vi "Func-엑셀 데이터를 그래프로 출력.vi"() -> ()   [LabVIEW 2015] (continued)
\t33.031\n30.25\t29.31\t33.06\n30.333\t29.34\t33.08\n30.417\t29.38\t33.1\n30.5\t29.41\t33.128\n30.583\t29.44\t33.149\n30.667\t29.49\t33.181\n30.75\t29.52\t33.201\n30.833\t29.58\t33.234\n30.917\t29.64\t33.257\n31\t29.69\t33.277\n31.083\t29.76\t33.311\n31.167\t29.83\t33.344\n31.25\t29.9\t33.378\n31.333\t29.99\t33.4\n31.417\t30.07\t33.435\n31.5\t30.16\t33.464\n31.583\t30.25\t33.499\n31.667\t30.34\t33.531\n31.75\t30.43\t33.566\n31.833\t30.52\t33.598\n31.917\t30.61\t33.637\n32\t30.7\t33.664\n32.083\t30.78\t33.702\n32.167\t30.87\t33.738\n32.25\t30.96\t33.777\n32.333\t31.05\t33.805\n32.417\t31.14\t33.841\n32.5\t31.22\t33.877\n32.583\t31.31\t33.921\n32.667\t31.39\t33.946\n32.75\t31.48\t33.992\n32.833\t31.56\t34.028\n32.917\t31.64\t34.072\n33\t31.72\t34.12\n33.083\t31.8\t34.156\n33.167\t31.89\t34.186\n33.25\t31.96\t34.234\n33.333\t32.04\t34.273\n33.417\t32.13\t34.311\n33.5\t32.21\t34.349\n33.583\t32.29\t34.399\n33.667\t32.38\t34.444\n33.75\t32.46\t34.48\n33.833\t32.54\t34.524\n33.917\t32.62\t34.567\n34\t32.7\t34.611\n34.083\t32.78\t34.659\n34.167\t32.86\t34.71\n34.25\t32.95\t34.745\n34.333\t33.03\t34.793\n34.417\t33.1\t34.843\n34.5\t33.19\t34.884\n34.583\t33.27\t34.936\n34.667\t33.34\t34.972\n34.75\t33.43\t35.024\n34.833\t33.51\t35.072\n34.917\t33.6\t35.12\n35\t33.68\t35.169\n35.083\t33.76\t35.219\n35.167\t33.84\t35.261\n35.25\t33.91\t35.317\n35.333\t34\t35.361\n35.417\t34.08\t35.414\n35.5\t34.16\t35.466\n35.583\t34.24\t35.516\n35.667\t34.32\t35.568\n35.75\t34.4\t35.617\n35.833\t34.48\t35.672\n35.917\t34.56\t35.721\n36\t34.64\t35.772\n36.083\t34.72\t35.825\n36.167\t34.81\t35.89\n36.25\t34.91\t35.929\n36.333\t34.98\t35.979\n36.417\t35.06\t36.035\n36.5\t35.15\t36.089\n36.583\t35.23\t36.138\n36.667\t35.31\t36.195\n36.75\t35.4\t36.259\n36.833\t35.47\t36.321\n36.917\t35.56\t36.369\n37\t35.64\t36.425\n37.083\t35.72\t36.47\n37.167\t35.81\t36.541\n37.25\t35.89\t36.585\n37.333\t35.96\t36.646\n37.417\t36.05\t36.697\n37.5\t36.13\t36.768\n37.583\t36.21\t36.809\n37.667\t36.3\t36.873\n37.75\t36.37\t36.934\n37.833\t36.46\t36.986\n37.917\t36.54\t37.046\n38\t36.62\t37.108\n38.083\t36.71\t37.157\n38.167\t36.79\t37.223\n38.25\t36.87\t37.283\n38.333\t36.96\t37.336\n38.417\t37.05\t37.39\n38.5\t37.13\t37.46\n38.583\t37.21\t37.511\n38.667\t37.3\t37.579\n38.75\t37.38\t37.633\n38.833\t37.47\t37.689\n38.917\t37.53\t37.751\n39\t37.62\t37.814\n39.083\t37.7\t37.879\n39.167\t37.78\t37.939\n39.25\t37.86\t37.999\n39.333\t37.95\t38.054\n39.417\t38.04\t38.114\n39.5\t38.1\t38.175\n39.583\t38.15\t38.25\n39.667\t38.2\t38.307\n39.75\t38.23\t38.366\n39.833\t38.28\t38.422\n39.917\t38.32\t38.477\n40\t38.4\t38.551\n40.083\t38.46\t38.614\n40.167\t38.52\t38.675\n40.25\t38.6\t38.739\n40.333\t38.69\t38.802\n40.417\t38.76\t38.873\n40.5\t38.85\t38.934\n40.583\t38.94\t39.002\n40.667\t39.03\t39.057\n40.75\t39.11\t39.12\n40.833\t39.2\t39.192\n40.917\t39.3\t39.243\n41\t39.39\t39.309\n41.083\t39.49\t39.369\n41.167\t39.58\t39.443\n41.25\t39.66\t39.511\n41.333\t39.74\t39.568\n41.417\t39.82\t39.634\n41.5\t39.91\t39.696\n41.583\t40.01\t39.763\n41.667\t40.1\t39.828\n41.75\t40.19\t39.893\n41.833\t40.27\t39.952\n41.917\t40.36\t40.023\n42\t40.44\t40.088\n42.083\t40.52\t40.146\n42.167\t40.61\t40.223\n42.25\t40.68\t40.279\n42.333\t40.76\t40.346\n42.417\t40.85\t40.417\n42.5\t40.93\t40.475\n42.583\t41.01\t40.548\n42.667\t41.09\t40.606\n42.75\t41.16\t40.673\n42.833\t41.24\t40.749\n42.917\t41.33\t40.807\n43\t41.42\t40.88\n43.083\t41.49\t40.941\n43.167\t41.57\t41.002\n43.25\t41.64\t41.07\n43.333\t41.72\t41.145\n43.417\t41.8\t41.199\n43.5\t41.89\t41.264\n43.583\t41.98\t41.344\n43.667\t42.06\t41.402\n43.75\t42.14\t41.472\n43.833\t42.22\t41.54\n43.917\t42.3\t41.604\n44\t42.38\t41.674\n44.083\t42.46\t41.753\n44.167\t42.55\t41.811\n44.25\t42.63\t41.88\n44.333\t42.71\t41.957\n44.417\t42.79\t42.015\n44.5\t42.88\t42.095\n44.583\t42.95\t42.158\n44.667\t43.04\t42.223\n44.75\t43.12\t42.29\n44.833\t43.21\t42.359\n45\t43.27\t42.427\n45\t43.27\t42.43\n45\t43.28\t42.439\n45\t43.29\t42.442\n45\t43.3\t42.448\n45\t43.3\t42.455\n45\t43.31\t42.461\n45\t43.31\t42.466\n45\t43.32\t42.471\n45\t43.33\t42.475\n45\t43.34\t42.483\n45\t43.35\t42.492\n45\t43.36\t42.497\n45\t43.36\t42.503\n45\t43.37\t42.512\n45\t43.38\t42.522\n45\t43.39\t42.525\n45\t43.39\t42.534\n45\t43.4\t42.54\n45\t43.41\t42.546\n45\t43.42\t42.554\n45\t43.43\t42.557\n45\t43.44\t42.568\n45\t43.44\t42.58\n45\t43.45\t42.586\n45\t43.46\t42.594\n45\t43.47\t42.6\n45\t43.48\t42.608\n45\t43.49\t42.612\n45\t43.5\t42.619\n45\t43.5\t42.627\n45\t43.51\t42.635\n45\t43.52\t42.642\n45\t43.53\t42.647\n45\t43.54\t42.654\n45\t43.55\t42.662\n45\t43.55\t42.668\n45\t43.56\t42.674\n45\t43.57\t42.682\n45\t43.58\t42.691\n45\t43.59\t42.698\n45\t43.59\t42.702\n45\t43.6\t42.705\n45\t43.61\t42.714\n45\t43.62\t42.719\n45\t43.62\t42.725\n45\t43.63\t42.73\n45\t43.64\t42.737\n45\t43.64\t42.747\n45\t43.65\t42.757\n45\t43.66\t42.763\n45\t43.67\t42.766\n45\t43.67\t42.776\n45\t43.68\t42.781\n45\t43.69\t42.787\n45\t43.69\t42.793\n45\t43.69\t42.802\n45\t43.7\t42.813\n45\t43.71\t42.827\n45\t43.72\t42.833\n45\t43.73\t42.839\n45\t43.73\t42.846\n45\t43.74\t42.851\n45\t43.75\t42.856\n45\t43.75\t42.86\n45\t43.76\t42.869\n45\t43.77\t42.874\n45\t43.78\t42.882\n45\t43.78\t42.888\n45\t43.78\t42.891\n45\t43.79\t42.897\n45\t43.8\t42.902\n45\t43.8\t42.915\n45\t43.81\t42.923\n45\t43.82\t42.93\n45\t43.83\t42.945\n45\t43.84\t42.953\n45\t43.84\t42.959\n45\t43.85\t42.963\n45\t43.86\t42.968\n45\t43.86\t42.975\n45\t43.86\t42.978\n45\t43.87\t42.982\n45\t43.88\t42.984\n45\t43.88\t42.997\n45\t43.88\t43.002\n45\t43.89\t43.011\n45\t43.9\t43.02\n45\t43.9\t43.025\n45\t43.91\t43.035\n45\t43.92\t43.042\n45\t43.92\t43.049\n45\t43.93\t43.052\n45\t43.93\t43.059\n45\t43.94\t43.068\n45\t43.95\t43.074\n45\t43.95\t43.08\n45\t43.96\t43.086\n45\t43.97\t43.089\n45\t43.97\t43.102\n45\t43.97\t43.104\n45\t43.98\t43.112\n45\t43.99\t43.119\n45\t43.99\t43.124\n45\t44\t43.135\n45\t44.01\t43.141\n45\t44.01\t43.153\n45\t44.02\t43.163\n45\t44.03\t43.171\n45\t44.03\t43.179\n45\t44.04\t43.189\n45\t44.05\t43.189\n45\t44.06\t43.191\n45\t44.06\t43.196\n45\t44.06\t43.203\n45\t44.06\t43.208\n45\t44.07\t43.214\n45\t44.07\t43.225\n45\t44.08\t43.229\n45\t44.08\t43.237\n45\t44.09\t43.239\n45\t44.09\t43.242\n45\t44.1\t43.254\n45\t44.1\t43.259\n45\t44.11\t43.266\n45\t44.12\t43.275\n45\t44.12\t43.286\n45\t44.13\t43.295\n45\t44.13\t43.299\n45\t44.14\t43.302\n45\t44.15\t43.31\n45\t44.15\t43.321\n45\t44.16\t43.325\n45\t44.16\t43.333\n45\t44.16\t43.342\n45\t44.16\t43.35\n45\t44.17\t43.362\n45\t44.17\t43.364\n45\t44.17\t43.371\n45\t44.18\t43.379\n45\t44.19\t43.384\n45\t44.19\t43.393\n45\t44.2\t43.398\n45\t44.2\t43.409\n45\t44.21\t43.413\n45\t44.21\t43.422\n45\t44.21\t43.425\n45\t44.22\t43.429\n45\t44.22\t43.434\n45\t44.22\t43.435\n45\t44.23\t43.441\n45\t44.23\t43.451\n45\t44.24\t43.46\n45\t44.24\t43.468\n45\t44.25\t43.478\n45\t44.26\t43.485\n45\t44.26\t43.492\n45\t44.26\t43.496\n45\t44.26\t43.502\n45\t44.27\t43.51\n45\t44.27\t43.521\n45\t44.28\t43.527\n45\t44.28\t43.533\n45\t44.29\t43.546\n45\t44.29\t43.55\n45\t44.3\t43.561\n45\t44.3\t43.565\n45\t44.31\t43.575\n45\t44.31\t43.592\n45\t44.32\t43.596\n45\t44.33\t43.605\n45\t44.33\t43.609\n45\t44.33\t43.617\n45\t44.34\t43.618\n45\t44.34\t43.618\n45\t44.35\t43.628\n45\t44.35\t43.633\n45\t44.35\t43.645\n45\t44.35\t43.65\n45\t44.36\t43.657\n45\t44.37\t43.67\n45\t44.37\t43.675\n45\t44.38\t43.683\n45\t44.38\t43.689\n45\t44.39\t43.696\n45\t44.39\t43.705\n45\t44.39\t43.714\n45\t44.4\t43.719\n45\t44.4\t43.724\n45\t44.41\t43.732\n45\t44.42\t43.739\n45\t44.42\t43.744\n45\t44.43\t43.753\n45\t44.43\t43.76\n45\t44.44\t43.765\n45\t44.44\t43.771\n45\t44.44\t43.777\n45\t44.45\t43.784\n45\t44.45\t43.786\n45\t44.45\t43.791\n45\t44.45\t43.797\n45\t44.46\t43.81\n45\t44.46\t43.817\n45\t44.47\t43.824\n45\t44.47\t43.832\n45\t44.48\t43.839\n45\t44.48\t43.846\n45\t44.48\t43.854\n45\t44.49\t43.857\n45\t44.49\t43.864\n45\t44.5\t43.871\n45\t44.5\t43.879\n45\t44.51\t43.888\n45\t44.51\t43.894\n45\t44.52\t43.9\n45\t44.52\t43.91\n45\t44.53\t43.916\n45\t44.53\t43.924\n45\t44.53\t43.933\n45\t44.53\t43.935\n45\t44.54\t43.939\n45\t44.54\t43.948\n45\t44.54\t43.954\n45\t44.54\t43.956\n45\t44.54\t43.964\n45\t44.55\t43.971\n45\t44.55\t43.98\n45\t44.55\t43.988\n45\t44.55\t43.995\n45\t44.56\t44.005\n45\t44.56\t44.015\n45\t44.57\t44.02\n45\t44.57\t44.025\n45\t44.57\t44.035\n45\t44.57\t44.038\n45\t44.58\t44.041\n45\t44.58\t44.05\n45\t44.59\t44.055\n45\t44.59\t44.064\n45\t44.59\t44.072\n45\t44.59\t44.083\n45\t44.6\t44.094\n45\t44.61\t44.101\n45\t44.61\t44.113\n45\t44.61\t44.122\n45\t44.62\t44.127\n45\t44.62\t44.131\n45\t44.62\t44.139\n45\t44.63\t44.144\n45\t44.63\t44.145\n45\t44.63\t44.158\n45\t44.64\t44.164\n45\t44.64\t44.171\n45\t44.64\t44.177\n45\t44.64\t44.179\n45\t44.64\t44.191\n45\t44.64\t44.193\n45\t44.64\t44.2\n45\t44.64\t44.205\n45\t44.65\t44.22\n45\t44.65\t44.224\n45\t44.66\t44.224\n45\t44.66\t44.233\n45\t44.67\t44.236\n45\t44.67\t44.244\n45\t44.67\t44.248\n45\t44.68\t44.259\n45\t44.68\t44.268\n45\t44.69\t44.278\n45\t44.69\t44.286\n45\t44.69\t44.293\n45\t44.7\t44.296\n45\t44.7\t44.302\n45\t44.7\t44.311\n45\t44.7\t44.316\n45\t44.7\t44.321\n45\t44.7\t44.323\n45\t44.71\t44.337\n45\t44.71\t44.343\n45\t44.71\t44.35\n45\t44.72\t44.356\n45\t44.72\t44.361\n45\t44.72\t44.375\n45\t44.72\t44.38\n45\t44.73\t44.388\n45\t44.73\t44.396\n45\t44.73\t44.402\n45\t44.73\t44.413\n45\t44.73\t44.417\n45\t44.73\t44.424\n45\t44.73\t44.429\n45\t44.73\t44.44\n45\t44.73\t44.446\n45\t44.74\t44.45\n45\t44.74\t44.463\n45\t44.74\t44.466\n45\t44.75\t44.469\n45\t44.75\t44.475\n45\t44.75\t44.482\n45\t44.76\t44.489\n45\t44.75\t44.492\n45\t44.76\t44.502\n45\t44.76\t44.513\n45\t44.76\t44.518\n45\t44.76\t44.522\n45\t44.77\t44.528\n45\t44.77\t44.533\n45\t44.78\t44.536\n45\t44.78\t44.54\n45\t44.78\t44.551\n45\t44.78\t44.556\n45\t44.78\t44.565\n45\t44.78\t44.577\n45\t44.79\t44.585\n45\t44.79\t44.598\n45\t44.79\t44.607\n45\t44.79\t44.614\n45\t44.79\t44.621\n45\t44.8\t44.628\n45\t44.8\t44.633\n45\t44.8\t44.638\n45\t44.8\t44.642\n45\t44.8\t44.648\n45\t44.81\t44.656\n45\t44.81\t44.663\n45\t44.81\t44.669\n45\t44.81\t44.677\n45\t44.81\t44.68\n45\t44.81\t44.688\n45\t44.81\t44.697\n45\t44.82\t44.704\n45\t44.82\t44.711\n45\t44.82\t44.724\n45\t44.82\t44.737\n45\t44.82\t44.743\n45\t44.82\t44.752\n45\t44.82\t44.755\n45\t44.82\t44.76\n45\t44.82\t44.762\n45\t44.82\t44.763\n45\t44.82\t44.77\n45\t44.83\t44.776\n45\t44.83\t44.779\n45\t44.83\t44.79\n45\t44.83\t44.798\n45\t44.83\t44.806\n45\t44.83\t44.816\n45\t44.83\t44.822\n45\t44.83\t44.832\n45\t44.83\t44.838\n45\t44.83\t44.841\n45\t44.83\t44.843\n45\t44.83\t44.848\n45\t44.83\t44.856\n45\t44.83\t44.859\n45\t44.84\t44.867\n45\t44.84\t44.875\n45\t44.84\t44.886\n45\t44.84\t44.893\n45\t44.85\t44.896\n45\t44.86\t44.908\n45\t44.87\t44.916\n45\t44.88\t44.925\n45\t44.89\t44.932\n45\t44.9\t44.942\n45\t44.91\t44.947\n45\t44.92\t44.951\n45\t44.93\t44.963\n45\t44.94\t44.966\n45\t44.95\t44.971\n45\t44.96\t44.98\n45\t44.97\t44.989\n45\t44.98\t45\n45\t45\t45\n45\t44.97\t45.005\n45\t44.97\t45.01\n45\t44.97\t45.015\n45\t44.97\t45.021\n45\t44.97\t45.025\n45\t44.97\t45.032\n45\t44.97\t45.038\n45\t44.97\t45.045\n45\t44.97\t45.053\n45\t44.97\t45.058\n45\t44.97\t45.066\n45\t44.97\t45.073\n45\t44.97\t45.079\n45\t44.97\t45.089\n45\t44.97\t45.093\n45\t44.97\t45.099\n45\t44.97\t45.108\n45\t44.97\t45.115\n45\t44.97\t45.121\n45\t44.97\t45.126\n45\t44.97\t45.132\n45\t44.97\t45.137\n45\t44.97\t45.145\n45\t44.98\t45.15\n45\t44.98\t45.156\n45\t44.98\t45.168\n45\t44.98\t45.174\n45\t44.98\t45.183\n45\t44.98\t45.189\n45\t44.98\t45.196\n45\t44.98\t45.201\n45\t44.98\t45.208\n45\t44.98\t45.214\n45\t44.98\t45.223\n45\t44.98\t45.229\n45\t44.98\t45.234\n45\t44.98\t45.243\n45\t44.98\t45.248\n45\t44.98\t45.25\n45\t44.98\t45.259\n45\t44.98\t45.265\n45\t44.98\t45.273\n45\t44.98\t45.283\n45\t44.98\t45.288\n45\t44.98\t45.299\n45\t44.98\t45.305\n45\t44.98\t45.313\n45\t44.98\t45.315\n45\t44.98\t45.327\n45\t44.98\t45.335\n45\t44.98\t45.339\n45\t44.98\t45.346\n45\t44.98\t45.35\n45\t44.98\t45.361\n45\t44.98\t45.363\n45\t45\t45.367\n45\t45\t45.377\n45\t45\t45.383\n45\t45\t45.388\n45\t45\t45.392\n45\t45\t45.399\n45\t45\t45.407\n45\t45\t45.414\n45\t45\t45.418\n45\t45\t45.423\n45\t45\t45.436\n45\t45\t45.441\n45\t45\t45.446\n45\t45\t45.456\n45\t45\t45.463\n45\t45\t45.47\n45\t45\t45.472\n45\t45\t45.478\n45\t45\t45.482\n45\t45\t45.489\n45\t45\t45.495\n45\t45\t45.501\n45\t45\t45.507\n45\t45\t45.514\n45\t45\t45.519\n45\t45\t45.526\n45\t45\t45.533\n45\t45\t45.539\n45\t45\t45.549\n45\t45\t45.554\n45\t45\t45.563\n45\t45\t45.571\n45\t45\t45.571\n45\t45\t45.577\n45\t45\t45.588\n45\t45\t45.597\n45\t45\t45.6\n45\t45\t45.61\n45\t45\t45.621\n45\t45\t45.628\n45\t45\t45.632\n45\t45\t45.636\n45\t45\t45.642\n45\t45\t45.647\n45\t45\t45.65\n45\t45\t45.653\n45\t45\t45.661\n45\t45\t45.667\n45\t45\t45.676\n45\t45\t45.682\n45\t45\t45.687\n45\t45\t45.695\n45\t45\t45.7\n45\t45\t45.707\n45\t45\t45.716\n45\t45\t45.724\n45\t45\t45.733\n45\t45\t45.743\n45\t45\t45.747\n45\t45\t45.754\n45\t45\t45.756\n45\t45\t45.761\n45\t45\t45.764\n45\t45\t45.769\n45\t45\t45.777\n45\t45\t45.782\n45\t45\t45.795\n45\t45\t45.8\n45\t45\t45.806\n45\t45\t45.814\n45\t45\t45.817\n45\t45\t45.818\n45\t45\t45.825\n45\t45\t45.832\n45\t45\t45.843\n45\t45\t45.85\n45\t45\t45.857\n45\t45\t45.868\n45\t45\t45.87\n45\t45\t45.875\n45\t45\t45.882\n45\t45\t45.889\n45\t45\t45.895\n45\t45\t45.903\n45\t45\t45.911\n45\t45\t45.917\n45\t45\t45.926\n45\t45\t45.93\n45\t45\t45.935\n45\t45\t45.939\n45\t45\t45.94\n45\t45\t45.946\n45\t45\t45.952\n45\t45\t45.957\n45\t45\t45.964\n45\t45\t45.973\n45\t45\t45.982\n45\t45\t45.987\n45\t45\t45.995\n45\t45\t45.999\n45\t45\t46.005\n45\t45\t46.013\n45\t45\t46.018\n45\t45\t46.024\n45\t45\t46.031\n45\t45\t46.039\n45\t45\t46.048\n45\t45\t46.052\n45\t45\t46.059\n45\t45\t46.068\n45\t45\t46.074\n45\t45\t46.076\n45\t45\t46.086\n45\t45\t46.091\n45\t45\t46.094\n45\t45\t46.098\n45\t45\t46.103\n45\t45\t46.111\n45\t45\t46.117\n45\t45\t46.122\n45\t45\t46.129\n45\t45\t46.14\n45\t45\t46.144\n45\t45\t46.151\n45\t45\t46.159\n45\t45\t46.169\n45\t45\t46.175\n45\t45\t46.18\n45\t45\t46.185\n45\t45\t46.189\n45\t45\t46.195\n45\t45\t46.199\n45\t45\t46.202\n45\t45\t46.209\n45\t45\t46.216\n45\t45\t46.224\n45\t45\t46.227\n45\t45\t46.229\n45\t45\t46.241\n45\t45\t46.249\n45\t45\t46.251\n45\t45\t46.258\n45\t45\t46.266\n45\t45\t46.27\n45\t45\t46.277\n45\t45\t46.277\n45\t45\t46.284\n45\t45\t46.289\n45\t45\t46.296\n45\t45\t46.304\n45\t45\t46.312\n45\t45\t46.319\n45\t45\t46.325\n45\t45\t46.338\n45\t45\t46.34\n45\t45\t46.347\n45\t45\t46.351\n45\t45\t46.356\n45\t45\t46.363\n45\t45\t46.368\n45\t45\t46.374\n45\t45\t46.383\n45\t45\t46.391\n45\t45\t46.396\n45\t45\t46.402\n45\t45\t46.404\n45\t45\t46.407\n45\t45\t46.412\n45\t45\t46.422\n45\t45\t46.43\n45\t45\t46.431\n45\t45\t46.439\n45\t45\t46.444\n45\t45\t46.446\n45\t45\t46.447\n45\t45\t46.451\n45\t45\t46.463\n45\t45\t46.467\n45\t45\t46.473\n45\t45\t46.482\n45\t45\t46.487\n45\t45\t46.489\n45\t45\t46.501\n45\t45\t46.505\n45\t45\t46.512\n45\t45\t46.522\n45\t45\t46.53\n45\t45\t46.536\n45\t45\t46.538\n45\t45\t46.545\n45\t45\t46.55\n45\t45\t46.554\n45\t45\t46.561\n45\t45\t46.57\n45\t45\t46.577\n45\t45\t46.583\n45\t45\t46.585\n45\t45\t46.597\n45\t45\t46.599\n45\t45\t46.602\n45\t45\t46.61\n45\t45\t46.616\n45\t45\t46.627\n45\t45\t46.629\n45\t45\t46.633\n45\t45\t46.64\n45\t45\t46.641\n45\t45\t46.646\n45\t45\t46.653\n45\t45\t46.657\n45\t45\t46.664\n45\t45\t46.671\n45\t45\t46.676\n45\t45\t46.679\n45\t45\t46.683\n45\t45\t46.692\n45\t45\t46.695\n45\t45\t46.704\n45\t45\t46.715\n45\t45\t46.718\n45\t45\t46.722\n45\t45\t46.725\n45\t45\t46.731\n45\t45\t46.734\n45\t45\t46.738\n45\t45\t46.745\n45\t45\t46.755\n45\t45\t46.759\n45\t45\t46.766\n45\t45\t46.775\n45\t45\t46.777\n45\t45\t46.781\n45\t45\t46.788\n45\t45\t46.793\n45\t45\t46.793\n45\t45\t46.799\n45\t45\t46.805\n45\t45\t46.811\n45\t45\t46.814\n45\t45\t46.819\n45\t45\t46.829\n45\t45\t46.834\n45\t45\t46.838\n45\t45\t46.845\n45\t45\t46.848\n45\t45\t46.857\n45\t45\t46.86\n45\t45\t46.869\n45\t45\t46.877\n45\t45\t46.885\n45\t45\t46.893\n45\t45\t46.896\n45\t45\t46.904\n45\t45\t46.906\n45\t45\t46.914\n45\t45\t46.923\n45\t45\t46.927\n45\t45\t46.934\n45\t45\t46.943\n45\t45\t46.95\n45\t45\t46.954\n45\t45\t46.959\n45\t45\t46.967\n45\t45\t46.971\n45\t45\t46.976\n45\t45\t46.978\n45\t45\t46.98\n45\t45\t46.985\n45\t45\t46.987\n45\t45\t46.992\n45\t45\t46.998\n45\t45\t47.007\n45\t45\t47.018\n45\t45\t47.022\n45\t45\t47.029\n45\t45\t47.031\n45\t45\t47.036\n45\t45\t47.043\n45\t45\t47.045\n45\t45\t47.048\n45\t45\t47.051\n45\t45\t47.064\n45\t45\t47.067\n45\t45\t47.066\n45\t45\t47.074\n45\t45\t47.08\n45\t45\t47.085\n45\t45\t47.091\n45\t45\t47.096\n45\t45\t47.103\n45\t45\t47.11\n45\t45\t47.115\n45\t45\t47.12\n45\t45\t47.123\n45\t45\t47.126\n45\t45\t47.13\n45\t45\t47.137\n45\t45\t47.142\n45\t45\t47.146\n45\t45\t47.155\n45\t45\t47.165\n45\t45\t47.169\n45\t45\t47.175\n45\t45\t47.179\n45\t45\t47.189\n45\t45\t47.19\n45\t45\t47.19\n45\t45\t47.194\n45\t45\t47.201\n45\t45\t47.206\n45\t45\t47.209\n45\t45\t47.219\n45\t45\t47.225\n45\t45\t47.233\n45\t45\t47.236\n45\t45\t47.241\n45\t45\t47.246\n45\t45\t47.251\n45\t45\t47.255\n45\t45\t47.259\n45\t45\t47.266\n45\t45\t47.269\n45\t45\t47.28\n45\t45\t47.28\n45\t45\t47.29\n45\t45\t47.297\n45\t45\t47.297\n45\t45\t47.302\n45\t45\t47.306\n45\t45\t47.311\n45\t45\t47.314\n45\t45\t47.323\n45\t45\t47.329\n45\t45\t47.334\n45\t45\t47.338\n45\t45\t47.343\n45\t45\t47.352\n45\t45\t47.352\n45\t45\t47.356\n45\t45\t47.368\n45\t45\t47.37\n45\t45\t47.371\n45\t45\t47.378\n45\t45\t47.381\n45\t45\t47.387\n45\t45\t47.389\n45\t45\t47.393\n45\t45\t47.402\n45\t45\t47.408\n45\t45\t47.41\n45\t45\t47.415\n45\t45\t47.421\n45\t45\t47.426\n45\t45\t47.431\n45\t45\t47.437\n45\t45\t47.446\n45\t45\t47.451\n45\t45\t47.461\n45\t45\t47.467\n45\t45\t47.468\n45\t45\t47.471\n45\t45\t47.475\n45\t45\t47.48\n45\t45\t47.489\n45\t45\t47.493\n45\t45\t47.499\n45\t45\t47.505\n45\t45\t47.511\n45\t45\t47.515\n45\t45\t47.516\n45\t45\t47.522\n45\t45\t47.53\n45\t45\t47.535\n45\t45\t47.54\n45\t45\t47.548\n45\t45\t47.549\n45\t45\t47.556\n45\t45\t47.561\n45\t45\t47.564\n45\t45\t47.569\n45\t45\t47.575\n45\t45\t47.58\n45\t45\t47.584\n45\t45\t47.589\n45\t45\t47.595\n45\t45\t47.596\n45\t45\t47.598\n45\t45\t47.603\n45\t45\t47.606\n45\t45\t47.613\n45\t45\t47.618\n45\t45\t47.627\n45\t45\t47.634\n45\t45\t47.638\n45\t45\t47.64\n45\t45\t47.64\n45\t45\t47.644\n45\t45\t47.65\n45\t45\t47.653\n45\t45\t47.664\n45\t45\t47.671\n45\t45\t47.675\n45\t45\t47.679\n45\t45\t47.686\n45\t45\t47.687\n45\t45\t47.687\n45\t45\t47.696\n45\t45\t47.702\n45\t45\t47.711\n45\t45\t47.717\n45\t45\t47.723\n45\t45\t47.731\n45\t45\t47.736\n45\t45\t47.739\n45\t45\t47.741\n45\t45\t47.745\n45\t45\t47.746\n45\t45\t47.747\n45\t45\t47.753\n45\t45\t47.756\n45\t45\t47.761\n45\t45\t47.769\n45\t45\t47.776\n45\t45\t47.78\n45\t45\t47.783\n45\t45\t47.79\n45\t45\t47.794\n45\t45\t47.798\n45\t45\t47.805\n45\t45\t47.813\n45\t45\t47.817\n45\t45\t47.819\n45\t45\t47.824\n45\t45\t47.825\n45\t45\t47.827\n45\t45\t47.832\n45\t45\t47.836\n45\t45\t47.843\n45\t45\t47.851\n45\t45\t47.857\n45\t45\t47.862\n45\t45\t47.868\n45\t45\t47.872\n45\t45\t47.873\n45\t45\t47.876\n45\t45\t47.879\n45\t45\t47.88\n45\t45\t47.882\n45\t45\t47.888\n45\t45\t47.893\n45\t45\t47.9\n45\t45\t47.905\n45\t45\t47.911\n45\t45\t47.915\n45\t45\t47.92\n45\t45\t47.921\n45\t45\t47.927\n45\t45\t47.929\n45\t45\t47.934\n45\t45\t47.945\n45\t45\t47.946\n45\t45\t47.953\n45\t45\t47.957\n45\t45\t47.966\n45\t45\t47.968\n45\t45\t47.966\n45\t45\t47.973\n45\t45\t47.979\n45\t45\t47.988\n45\t45\t47.987\n45\t45\t47.995\n45\t45\t48.003\n45\t45\t48.006\n45\t45\t48.01\n45\t45\t48.009\n45\t45\t48.015\n45\t45\t48.021\n45\t45\t48.028\n45\t45\t48.029\n45\t45\t48.035\n45\t45\t48.041\n45\t45\t48.042\n45\t45\t48.051\n45\t45\t48.054\n45\t45\t48.062\n45\t45\t48.067\n45\t45\t48.071\n45\t45\t48.078\n45\t45\t48.08\n45\t45\t48.081\n45\t45\t48.084\n45\t45\t48.09\n45\t45\t48.094\n45\t45\t48.099\n45\t45\t48.105\n45\t45\t48.109\n45\t45\t48.114\n45\t45\t48.12\n45\t45\t48.121\n45\t45\t48.125\n45\t45\t48.129\n45\t45\t48.13\n45\t45\t48.133\n45\t45\t48.141\n45\t45\t48.147\n45\t45\t48.153\n
